vi "Create Trigger Model Constant Limit Branch.vi"(0 "VISA resource name":refnum<visa-resource-name>, 1 "Limit B":dbl, 2 "Measurement Block":i32=1 min=1 format="%#.6g", 5 "Block Number (1)":i32=1 min=1 format="%#.6g", 7 "Limit Type":u16(ring) items=["Above", "Below", "Inside", "Outside"], 9 "Limit A":dbl, 11 "error in (no error)":errorcluster, 12 "Branch To Block":i32=1 min=1 format="%#.6g") -> (4 "VISA resource name out":refnum<visa-resource-name>, 15 "error out":errorcluster)   [LabVIEW 2018, in "Keithley DMM7512.lvlib"]
doc: "This VI defines a trigger model block that branches to a block outside the normal trigger model flow if a measurement meets preset criteria."
uses:
  <instrlib>/Keithley DMM7512/Keithley DMM7512.lvlib
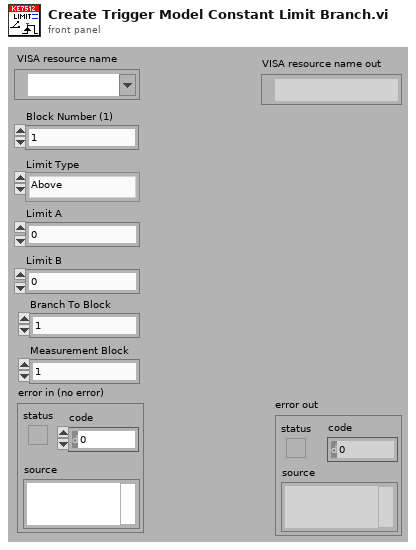
[diagram p1: front panel]
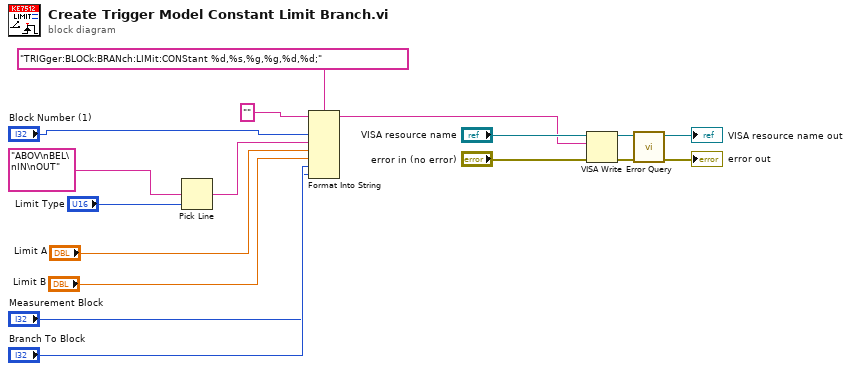
[diagram p0: block diagram]
diagram:
  n1 = Pick Line(multi-line string="ABOV\nBEL\nIN\nOUT", line index="Limit Type") -> (output string=w7:string)  [unwired: 1 in]
  n2 = Format Into String(format string="TRIGger:BLOCk:BRANch:LIMit:CONStant %d,%s,%g,%g,%d,%d;", initial string="", "Block Number (1)", w7, "Limit A", "Limit B", "Branch To Block", "Measurement Block") -> (resulting string=w9:string)  [unwired: 1 in, 1 out]
  n3 = VISA Write(VISA resource name="VISA resource name", write buffer=w9, error in (no error)="error in (no error)") -> (VISA resource name out=w13:refnum<visa-resource-name>, error out=w12:errorcluster)  [unwired: 1 out]
  n4 = call <instrlib>:"Error Query.vi"("error in (no error)"=w12, "VISA resource name"=w13) -> ("error out"=→"error out":errorcluster, "VISA resource name out"=→"VISA resource name out":refnum<visa-resource-name>)  [unwired: 8 out]
